vi "calc exptime diff.vi"(8 "error in (no error)":errorcluster, 10 "ACS mode":u16(ring), 11 "Simulated_CCD_Camera in":refnum<class "Sim_CCD.lvclass">) -> (0 "error out":errorcluster, 2 "effective exptime":dbl, 3 "Simulated_CCD_Camera out":refnum<class "Sim_CCD.lvclass">)   [LabVIEW 2018, in "Sim_CCD.lvclass"]
uses:
  Sim_CCD.lvclass
  Sim_CCD.lvclass/Sim_CCD.ctl
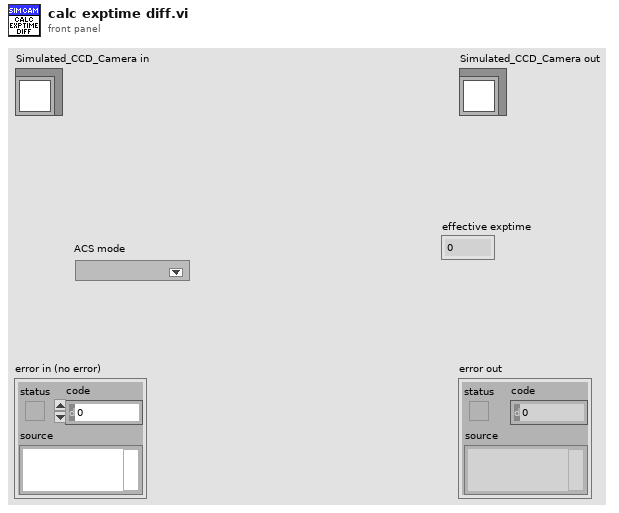
[diagram p1: front panel]
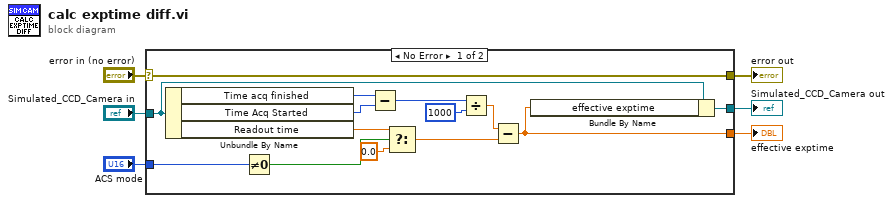
[diagram p0: block diagram]
diagram:
  n1 = case shown="No Error" "error in (no error)" {
    selector: "error in (no error)" -> [w8 w22]
    tunnel: [w8 w22] -> w5
    tunnel: [w9 w21] -> w3
    tunnel: "Simulated_CCD_Camera in" -> [w10 w21]
    tunnel: "ACS mode" -> [w11 _]
    tunnel: [w7 _] -> w1
    frame No Error {
      n2 = Unbundle By Name(w10) -> ("Time acq finished"=w20:u32, "Time Acq Started"=w19:u32, "Readout time"=w15:dbl)
      n3 = Not Equal To 0?(x=w11) -> (x != 0?=w12:bool)
      n4 = Subtract(x=w20, y=w19) -> (x-y=w18:u32)
      n5 = Select(t=w15, s=w12, f=0.0) -> (s? t:f=w13:dbl)
      n6 = Divide(x=w18, y=1000) -> (x/y=w16:dbl)
      n7 = Subtract(x=w16, y=w13) -> (x-y=w7:dbl)
      n8 = Bundle By Name(cluster=w10, "effective exptime"=w7) -> (w9:refnum<class "Sim_CCD.lvclass">)
    }
    frame Error {
    }
  }
  "error out" <- w5
  "Simulated_CCD_Camera out" <- w3
  "effective exptime" <- w1
